vi "galvanic.vi"(4 "Data Input":T1 {"Data Channels" format="%.2f"}, 7 "loaded filename":path) -> ()   [LabVIEW 2013]
panel:
  out "neg edges":i32[](array[numeric])
  out "pos edges":i32[](array[numeric])
  in  "Quadrant size from edge (sec)":dbl=10.0
  in  "Threshold":dbl=300.0 format="%.2f"
  in  "Start":bool
  in  "Trigger Channel (Other)":u16(ring)=25 items=["Hx Position-in-Head", "Hy Position-in-Head", "Hz Position-in-Head", "Hx Velocity-in-Head", "Hy Velocity-in-Head", "Hz Velocity-in-Head", "Hl Velocity-in-Head", "Hr Velocity-in-Head", "Lx Position-in-Head", "Ly Position-in-Head", "Lz Position-in-Head", "Lx Velocity-in-Head", "Ly Velocity-in-Head", "Lz Velocity-in-Head", "Ll Velocity-in-Head", "Lr Velocity-in-Head", "Rx Position-in-Head", "Ry Position-in-Head", "Rz Position-in-Head", "Rx Velocity-in-Head", "Ry Velocity-in-Head", "Rz Velocity-in-Head", "Rl Velocity-in-Head", "Rr Velocity-in-Head", "Button", "Ascension X or ch25", "Ascension X Vel", "Ascension Y", "Ascension Y Vel", "Ascension Z", "Ascension q1", "Chair Position", "Chair Velocity", " "]
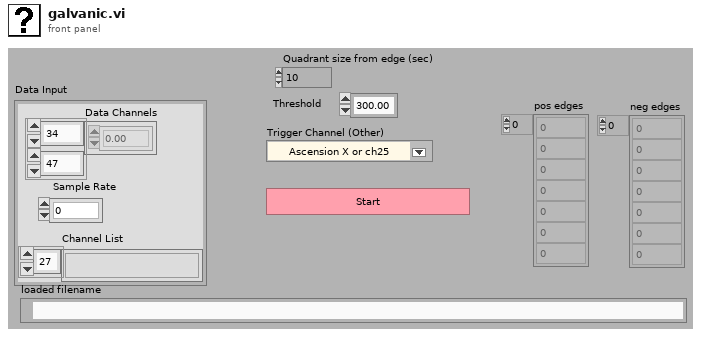
[diagram p1: front panel]
types:
  T1 = cluster{"Data Channels":dbl[][], "Sample Rate":i32, "Channel List":string[]}
  T2 = cluster{"Data Output":cluster{"Data Channels":dbl[][], "Sample Rate":i32, "Channel List":string[]}, "Impulse Positions":cluster{"Start":i32, "End":i32, "Impulse Plane":enum16{"Other", "Yaw", "Pitch", "Roll", "LARP", "RALP"}, "Impulse Direction +ve?":bool, "Time offset":i32, "Amplitude offset":dbl}[], "Old Impulse positions for Undo":cluster{"Start":i32, "End":i32, "Impulse Plane":enum16{"Other", "Yaw", "Pitch", "Roll", "LARP", "RALP"}, "Impulse Direction +ve?":bool, "Time offset":i32, "Amplitude offset":dbl}[], "No. Imp":i32}
  T3 = enum16{"open", "open or create", "create or replace", "create", "open (read only)"}
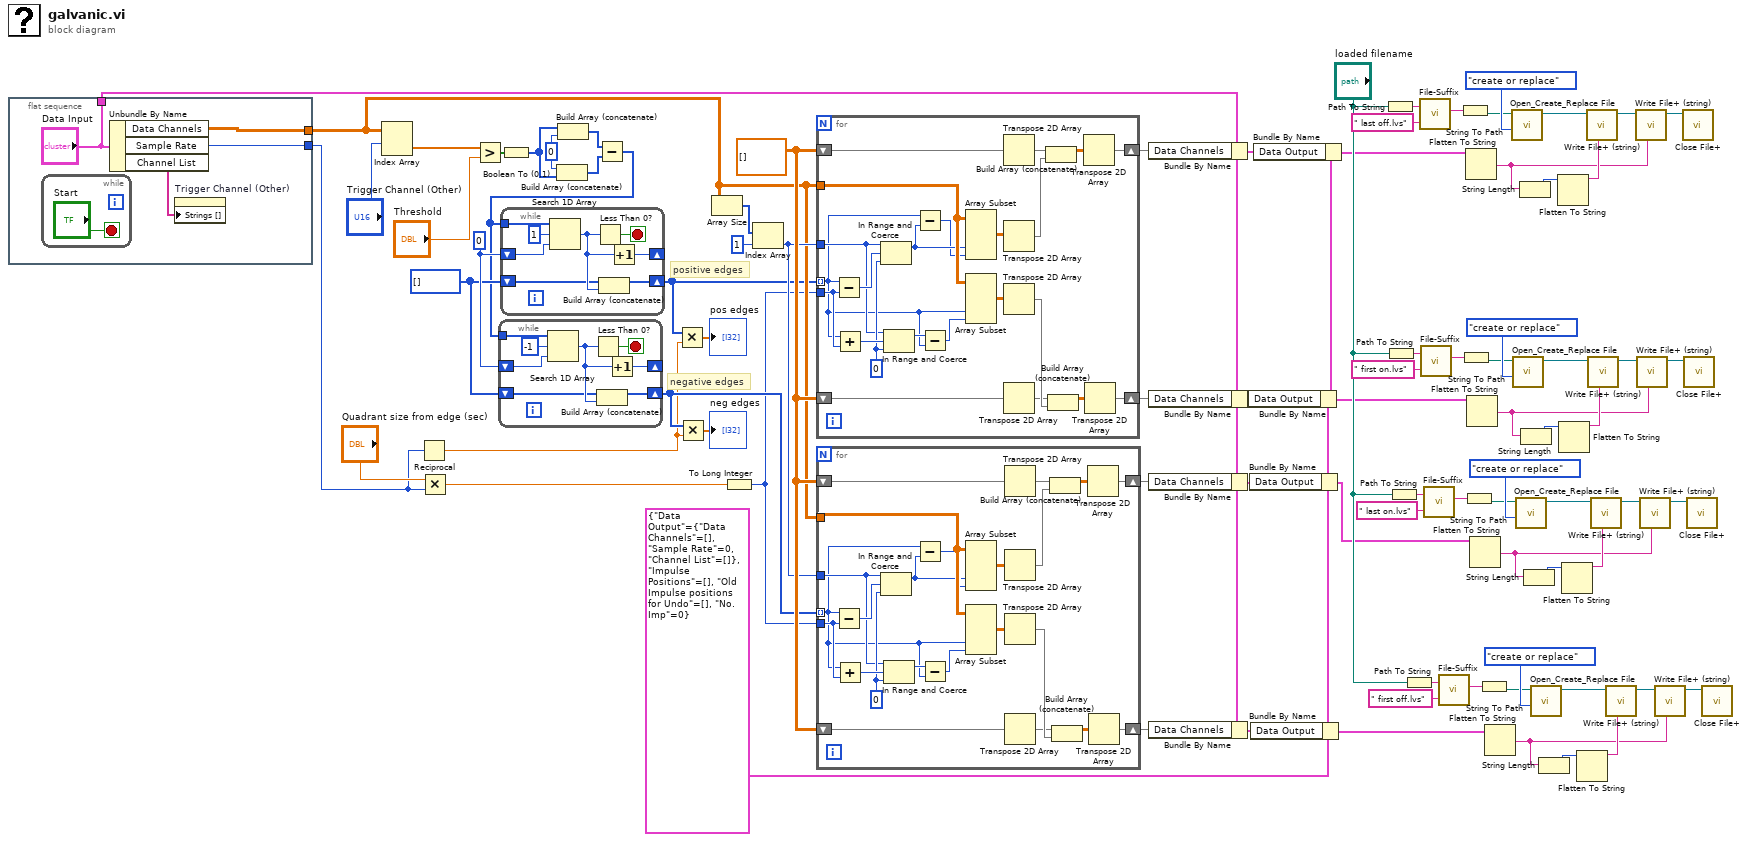
[diagram p0: block diagram]
diagram:
  w2 = T2 {"Data Output"={"Data Channels"=[], "Sample Rate"=0, "Channel List"=[]}, "Impulse Positions"=[], "Old Impulse positions for Undo"=[], "No. Imp"=0}
  w71 = dbl[][] []
  w75 = i32[] []
  w76 = 0
  w80 = 0
  # "negative edges"
  # "positive edges"
  n1 = flat-sequence {
    tunnel: [w88] -> w69
    tunnel: [w87] -> w10
    tunnel: ["Data Input"] -> w45
    frame #0 {
      n2 = while {
        stop <- "Start" stop-if-true
      }
      n3 = Unbundle By Name("Data Input") -> ("Data Channels"=w88:dbl[][], "Sample Rate"=w87:i32, "Channel List"=w85:string[])
      n4 = property on="Trigger Channel (Other)" class="Ring (strict)"("Strings []"=w85) -> ()  [unwired: 2 in, 2 out]
    }
  }
  n5 = Index Array(array=w69, index (row)="Trigger Channel (Other)") -> (element=w83:dbl[])  [unwired: 1 in]
  n6 = Reciprocal(x=w10) -> (1/x=w61:dbl)
  n7 = Multiply(x="Quadrant size from edge (sec)", y=w10) -> (x*y=w65:dbl)
  n8 = Greater?(x=w83, y="Threshold") -> (0:w81:bool[])
  n9 = Boolean To (0,1)(Boolean=w81) -> (0, 1=w77:i16[])
  n10 = Build Array (concatenate)(w80, w77) -> (w78:i32[])
  n11 = Build Array (concatenate)(w77, w80) -> (w79:i32[])
  n12 = Subtract(x=w79, y=w78) -> (x-y=w74:i32[])
  n13 = while {
    tunnel: w74 -> [w93]
    shift-right: [w90] -> _
    shift-left: w76 -> [w96]
    shift-right: [w92] -> w64
    shift-left: w75 -> [w91]
    stop <- w95 stop-if-true
    n14 = Search 1D Array(1D array=w93, element=-1, start index (0)=w96) -> (index of element=w94:i32)
    n15 = Less Than 0?(x=w94) -> (x < 0?=w95:bool)
    n16 = Build Array (concatenate)(w91, w94) -> (w92:i32[])
    n17 = Increment(x=w94) -> (x+1=w90:i32)
  }
  n18 = while {
    tunnel: w74 -> [w101]
    shift-right: [w98] -> _
    shift-left: w76 -> [w104]
    shift-right: [w100] -> w67
    shift-left: w75 -> [w99]
    stop <- w103 stop-if-true
    n19 = Search 1D Array(1D array=w101, element=1, start index (0)=w104) -> (index of element=w102:i32)
    n20 = Less Than 0?(x=w102) -> (x < 0?=w103:bool)
    n21 = Build Array (concatenate)(w99, w102) -> (w100:i32[])
    n22 = Increment(x=w102) -> (x+1=w98:i32)
  }
  n23 = Multiply(x=w67, y=w61) -> (x*y=→"pos edges":dbl[])
  n24 = Multiply(x=w64, y=w61) -> (x*y=→"neg edges":dbl[])
  n25 = Array Size(array=w69) -> (size(s)=w73:i32[])
  n26 = To Long Integer(number=w65) -> (32bit integer=w63:i32)
  n27 = Index Array(array=w73, index=1) -> (element=w70:i32)
  n28 = for {
    tunnel: w69 -> [w127]
    tunnel: w67 -> [w112] mode=indexing
    tunnel: w63 -> [w126]
    tunnel: w70 -> [w123]
    shift-right: [w107] -> w49
    shift-left: w71 -> [w119]
    shift-right: [w106] -> w48
    shift-left: w71 -> [w118]
    w124 = 0 ("lower limit")
    n29 = Subtract(x=w112, y=w126) -> (x-y=w128:i32)
    n30 = Add(x=w112, y=w126) -> (x+y=w125:i32)
    n31 = In Range and Coerce(upper limit=w123, x=w128, lower limit=w124) -> (coerced(x)=w115:i32)  [unwired: 1 out]
    n32 = In Range and Coerce(upper limit=w123, x=w125, lower limit=w124) -> (coerced(x)=w122:i32)  [unwired: 1 out]
    n33 = Subtract(x=w112, y=w115) -> (x-y=w114:i32)
    n34 = Subtract(x=w122, y=w112) -> (x-y=w113:i32)
    n35 = Array Subset(array=w127, index (col)=w115, length (col)=w114) -> (w121:dbl[][])  [unwired: 2 in]
    n36 = Array Subset(array=w127, index (col)=w112, length (col)=w113) -> (w117:dbl[][])  [unwired: 2 in]
    n37 = Transpose 2D Array(2D array=w119) -> (transposed array=w109:dbl[][])
    n38 = Transpose 2D Array(2D array=w121) -> (transposed array=w111:dbl[][])
    n39 = Transpose 2D Array(2D array=w117) -> (transposed array=w110:dbl[][])
    n40 = Transpose 2D Array(2D array=w118) -> (transposed array=w108:dbl[][])
    n41 = Build Array (concatenate)(w109, w111) -> (w120:dbl[][])
    n42 = Build Array (concatenate)(w108, w110) -> (w116:dbl[][])
    n43 = Transpose 2D Array(2D array=w120) -> (transposed array=w107:dbl[][])
    n44 = Transpose 2D Array(2D array=w116) -> (transposed array=w106:dbl[][])
  }
  n45 = for {
    tunnel: w69 -> [w150]
    tunnel: w64 -> [w135] mode=indexing
    tunnel: w63 -> [w149]
    tunnel: w70 -> [w146]
    shift-right: [w134] -> w47
    shift-left: w71 -> [w142]
    shift-right: [w133] -> w46
    shift-left: w71 -> [w141]
    w147 = 0 ("lower limit")
    n46 = Subtract(x=w135, y=w149) -> (x-y=w151:i32)
    n47 = Add(x=w135, y=w149) -> (x+y=w148:i32)
    n48 = In Range and Coerce(upper limit=w146, x=w151, lower limit=w147) -> (coerced(x)=w137:i32)  [unwired: 1 out]
    n49 = In Range and Coerce(upper limit=w146, x=w148, lower limit=w147) -> (coerced(x)=w145:i32)  [unwired: 1 out]
    n50 = Subtract(x=w135, y=w137) -> (x-y=w138:i32)
    n51 = Subtract(x=w145, y=w135) -> (x-y=w136:i32)
    n52 = Array Subset(array=w150, index (col)=w137, length (col)=w138) -> (w144:dbl[][])  [unwired: 2 in]
    n53 = Array Subset(array=w150, index (col)=w135, length (col)=w136) -> (w140:dbl[][])  [unwired: 2 in]
    n54 = Transpose 2D Array(2D array=w142) -> (transposed array=w129:dbl[][])
    n55 = Transpose 2D Array(2D array=w144) -> (transposed array=w132:dbl[][])
    n56 = Transpose 2D Array(2D array=w140) -> (transposed array=w131:dbl[][])
    n57 = Transpose 2D Array(2D array=w141) -> (transposed array=w130:dbl[][])
    n58 = Build Array (concatenate)(w129, w132) -> (w143:dbl[][])
    n59 = Build Array (concatenate)(w130, w131) -> (w139:dbl[][])
    n60 = Transpose 2D Array(2D array=w143) -> (transposed array=w134:dbl[][])
    n61 = Transpose 2D Array(2D array=w139) -> (transposed array=w133:dbl[][])
  }
  n62 = Bundle By Name(cluster=w45, "Data Channels"=w49) -> (w8:T1)
  n63 = Bundle By Name(cluster=w45, "Data Channels"=w48) -> (w7:T1)
  n64 = Bundle By Name(cluster=w45, "Data Channels"=w47) -> (w5:T1)
  n65 = Bundle By Name(cluster=w45, "Data Channels"=w46) -> (w3:T1)
  n66 = Bundle By Name(cluster=w2, "Data Output"=w7) -> (w6:T2)
  n67 = Bundle By Name(cluster=w2, "Data Output"=w5) -> (w4:T2)
  n68 = Bundle By Name(cluster=w2, "Data Output"=w3) -> (w1:T2)
  n69 = Bundle By Name(cluster=w2, "Data Output"=w8) -> (w9:T2)
  n70 = Path To String(path="loaded filename") -> (string=w52:string)
  n71 = Path To String(path="loaded filename") -> (string=w36:string)
  n72 = Path To String(path="loaded filename") -> (string=w25:string)
  n73 = Path To String(path="loaded filename") -> (string=w14:string)
  n74 = call "File-Suffix.vi"("Substring"=" last off.lvs", "String 2"=w52) -> ("String"=w50:string)
  n75 = call "File-Suffix.vi"("Substring"=" first on.lvs", "String 2"=w36) -> ("String"=w34:string)
  n76 = call "File-Suffix.vi"("Substring"=" last on.lvs", "String 2"=w25) -> ("String"=w23:string)
  n77 = call "File-Suffix.vi"("Substring"=" first off.lvs", "String 2"=w14) -> ("String"=w12:string)
  n78 = String To Path(string=w50) -> (path=w58:path)
  n79 = String To Path(string=w34) -> (path=w42:path)
  n80 = String To Path(string=w23) -> (path=w31:path)
  n81 = Flatten To String(anything=w9) -> (data string=w55:string)  [unwired: 3 in, 2 out]
  n82 = Flatten To String(anything=w6) -> (data string=w39:string)  [unwired: 3 in, 2 out]
  n83 = Flatten To String(anything=w4) -> (data string=w28:string)  [unwired: 3 in, 2 out]
  n84 = String To Path(string=w12) -> (path=w20:path)
  n85 = Flatten To String(anything=w1) -> (data string=w17:string)  [unwired: 3 in, 2 out]
  n86 = call <vilib>:"Open_Create_Replace File.vi"("function (open:0)"=T3."create or replace", "file path"=w58) -> ("refnum"=w53:refnum<file>)  [unwired: 6 in, 3 out]
  n87 = call <vilib>:"Open_Create_Replace File.vi"("function (open:0)"=T3."create or replace", "file path"=w42) -> ("refnum"=w37:refnum<file>)  [unwired: 6 in, 3 out]
  n88 = call <vilib>:"Open_Create_Replace File.vi"("function (open:0)"=T3."create or replace", "file path"=w31) -> ("refnum"=w26:refnum<file>)  [unwired: 6 in, 3 out]
  n89 = String Length(string=w55) -> (length=w57:i32)
  n90 = String Length(string=w39) -> (length=w41:i32)
  n91 = String Length(string=w28) -> (length=w30:i32)
  n92 = call <vilib>:"Open_Create_Replace File.vi"("function (open:0)"=T3."create or replace", "file path"=w20) -> ("refnum"=w15:refnum<file>)  [unwired: 6 in, 3 out]
  n93 = String Length(string=w17) -> (length=w19:i32)
  n94 = Flatten To String(anything=w57) -> (data string=w56:string)  [unwired: 3 in, 2 out]
  n95 = Flatten To String(anything=w41) -> (data string=w40:string)  [unwired: 3 in, 2 out]
  n96 = Flatten To String(anything=w30) -> (data string=w29:string)  [unwired: 3 in, 2 out]
  n97 = Flatten To String(anything=w19) -> (data string=w18:string)  [unwired: 3 in, 2 out]
  n98 = call <vilib>:"Write File+ (string).vi"("string"=w56, "refnum"=w53) -> ("dup refnum"=w54:refnum<file>)  [unwired: 5 in, 2 out]
  n99 = call <vilib>:"Write File+ (string).vi"("string"=w40, "refnum"=w37) -> ("dup refnum"=w38:refnum<file>)  [unwired: 5 in, 2 out]
  n100 = call <vilib>:"Write File+ (string).vi"("string"=w29, "refnum"=w26) -> ("dup refnum"=w27:refnum<file>)  [unwired: 5 in, 2 out]
  n101 = call <vilib>:"Write File+ (string).vi"("string"=w18, "refnum"=w15) -> ("dup refnum"=w16:refnum<file>)  [unwired: 5 in, 2 out]
  n102 = call <vilib>:"Write File+ (string).vi"("string"=w55, "refnum"=w54) -> ("dup refnum"=w60:refnum<file>)  [unwired: 5 in, 2 out]
  n103 = call <vilib>:"Write File+ (string).vi"("string"=w39, "refnum"=w38) -> ("dup refnum"=w44:refnum<file>)  [unwired: 5 in, 2 out]
  n104 = call <vilib>:"Write File+ (string).vi"("string"=w28, "refnum"=w27) -> ("dup refnum"=w33:refnum<file>)  [unwired: 5 in, 2 out]
  n105 = call <vilib>:"Write File+ (string).vi"("string"=w17, "refnum"=w16) -> ("dup refnum"=w22:refnum<file>)  [unwired: 5 in, 2 out]
  n106 = call <vilib>:"Close File+.vi"("refnum"=w60) -> ()  [unwired: 4 in, 3 out]
  n107 = call <vilib>:"Close File+.vi"("refnum"=w44) -> ()  [unwired: 4 in, 3 out]
  n108 = call <vilib>:"Close File+.vi"("refnum"=w33) -> ()  [unwired: 4 in, 3 out]
  n109 = call <vilib>:"Close File+.vi"("refnum"=w22) -> ()  [unwired: 4 in, 3 out]
